vi "Igor_ArraytoIgorWave.vi"   [LabVIEW 2019]
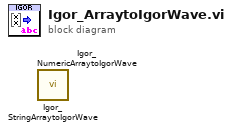
[diagram p0: block diagram]
diagram:
  n1 = call "Igor_StringArraytoIgorWave.vi"() -> ()  [unwired: 10 in, 2 out]
  n2 = call "Igor_NumericArraytoIgorWave.vi"() -> ()  [unwired: 10 in, 2 out]
